vi "07_Project_5_Temp_Control1.vi"() -> ()   [LabVIEW 2014]
panel:
  out "Data Details":string
  out "FAN":bool
  in  "Power":bool
  out "Current Temperature":dbl format="%#_2g"
  in  "On/Off":bool
  in  "Low Limit":dbl
  in  "High Limit":dbl
  out "Waveform Chart":cluster{"High Limit":dbl, "Low Limit":dbl, dbl}(graph)
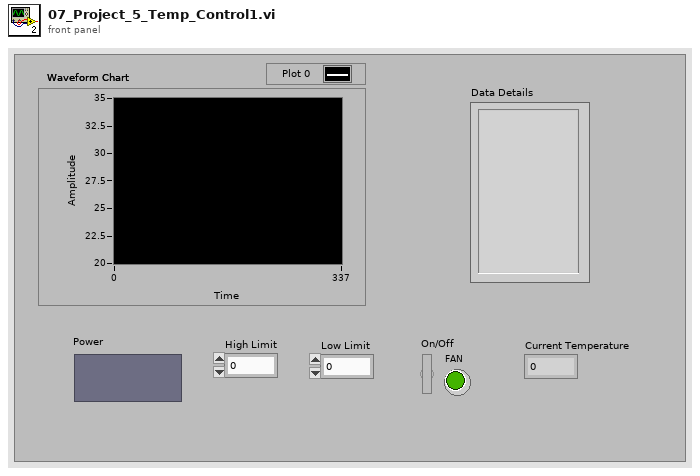
[diagram p1: front panel]
types:
  T1 = enum16{"open", "replace", "create", "open or create", "replace or create", "replace or create with confirmation"}
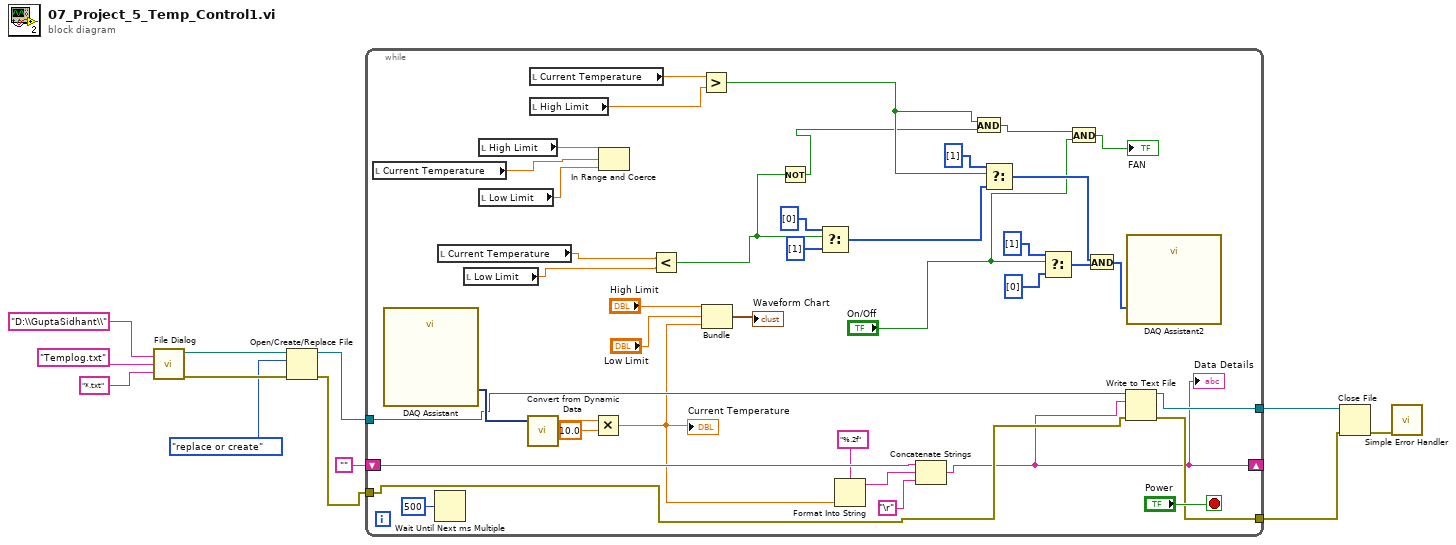
[diagram p0: block diagram]
diagram:
  n1 = call "File Dialog"("prompt"="D:\\GuptaSidhant\\", "default name"="Templog.txt", "pattern (all files)"="*.txt" ("pattern label")) -> ("selected path"=w8:path, "error out"=w9:errorcluster)  [unwired: 9 in, 2 out]
  n2 = Open/Create/Replace File(file path (use dialog)=w8, error in=w9, operation (0:open)=T1."replace or create") -> (refnum out=w1:refnum<file>, error out=w4:errorcluster)  [unwired: 3 in, 1 out]
  n3 = while {
    shift-right: [w26] -> _
    shift-left: "" -> [w44]
    tunnel: w4 -> [w27]
    tunnel: [w35] -> w3
    tunnel: [w36] -> w2
    tunnel: w1 -> [w34]
    stop <- "Power" stop-if-true
    n4 = local read "Current Temperature"() -> (w30:dbl)
    n5 = call "DAQ Assistant"() -> ("data"=w51:dynamicdata)  [unwired: 16 in, 3 out]
    n6 = Wait Until Next ms Multiple(millisecond multiple=u32 500) -> ()  [unwired: 1 out]
    n7 = local read "Current Temperature"() -> (w38:dbl)
    n8 = local read "Low Limit"() -> (w37:dbl)
    n9 = local read "High Limit"() -> (w32:dbl)
    n10 = local read "Low Limit"() -> (w31:dbl)
    n11 = call "Convert from Dynamic Data"("Dynamic Data Type"=w51) -> ("Scalar"=w47:dbl)  [unwired: 3 in]
    n12 = local read "Current Temperature"() -> (w39:dbl)
    n13 = local read "High Limit"() -> (w40:dbl)
    n14 = Multiply(x=w47, y=10.0) -> (x*y=w33:dbl)
    "Current Temperature" <- w33
    n15 = In Range and Coerce(upper limit=w32, x=w30, lower limit=w31) -> ()  [unwired: 2 out]
    n16 = Less?(x=w38, y=w37) -> (x < y?=w13:bool)
    n17 = Greater?(x=w39, y=w40) -> (0:w16:bool)
    n18 = Bundle("High Limit"="High Limit", "Low Limit"="Low Limit", w33) -> (→"Waveform Chart":cluster{"High Limit":dbl, "Low Limit":dbl, dbl})  [unwired: 1 in]
    n19 = Not(x=w13) -> (.not. x?=w14:bool)
    n20 = Select(t=u32[] [0] ("data"), s=w13, f=u32[] [1]) -> (s? t:f=w20:u32[])
    n21 = Format Into String(format string="%.2f", w33) -> (resulting string=w43:string)  [unwired: 2 in, 1 out]
    n22 = Concatenate Strings(w44, w43, "\r") -> (w26:string)
    "Data Details" <- w26
    n23 = And(x=w16, y=w14) -> (x .and. y?=w15:bool)
    n24 = Select(t=u32[] [1] ("data"), s=w16, f=w20) -> (s? t:f=w22:u32[])
    n25 = Select(t=u32[] [1] ("data"), s="On/Off", f=u32[] [0] ("data")) -> (s? t:f=w24:u32[])
    n26 = And(x=w15, y="On/Off") -> (x .and. y?=→"FAN":bool)
    n27 = And(x=w22, y=w24) -> (x .and. y?=w23:u32[])
    n28 = Write to Text File(file (use dialog)=w34, text=w26, error in=w27) -> (refnum out=w36:refnum<file>, error out=w35:errorcluster)  [unwired: 1 in, 1 out]
    n29 = call "DAQ Assistant2"("data"=w23) -> ()  [unwired: 17 in, 2 out]
  }
  n30 = Close File(refnum=w2, error in=w3) -> (error out=w6:errorcluster)  [unwired: 1 out]
  n31 = call <vilib>:"Simple Error Handler.vi"("error in (no error)"=w6) -> ()  [unwired: 4 in, 5 out]
